vi "T Test (mean).vi"(6 "alternative hypothesis":i32(ring) items=["mean(pop) != mean"=0, "mean(pop) > mean"=1, "mean(pop) < mean"=-1], 9 "significance level":dbl=0.05, 10 "mean":dbl, 11 "sample set":dbl[](array[numeric])) -> (0 "error":i32, 1 "confidence interval":cluster{"low":dbl, "high":dbl}={"low"=0.8260722090132093, "high"=0.8260722090132093} {"high" format="%.6g"; "low" format="%.6g"}, 2 "p value":dbl=0.05 format="%.6g", 3 "reject the null hypothesis":bool, 4 "t test info":T1 {"sample t value" format="%_6g"; "t value" format="%_6g"; "sample se mean" format="%_6g"; "sample std" format="%_6g"; "sample mean" format="%_6g"})   [LabVIEW 2017, in "NI_Gmath.lvlib"]
doc: "See pages 278+ from Applied Statistics and Probability for Engineers (Montgomery) - 3rd Edition."
uses:
  NI_Gmath.lvlib
  st_t_control.ctl
  NI_AALBase.lvlib
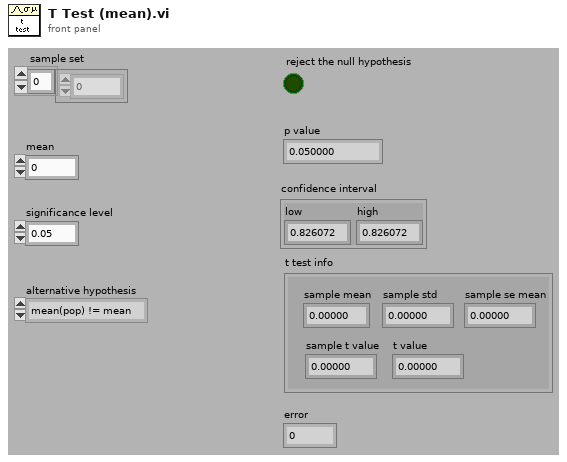
[diagram p1: front panel]
types:
  T1 = typedef "NI_Gmath.lvlib/st_t_control.ctl" = cluster{"sample mean":dbl, "sample std":dbl, "sample se mean":dbl, "sample t value":dbl, "t value":dbl}
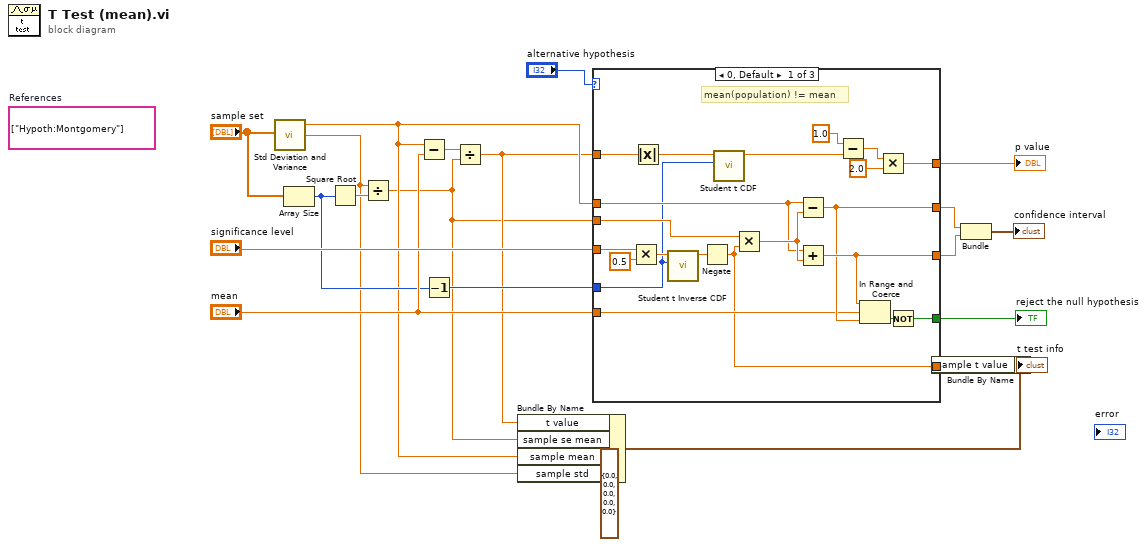
[diagram p0: block diagram]
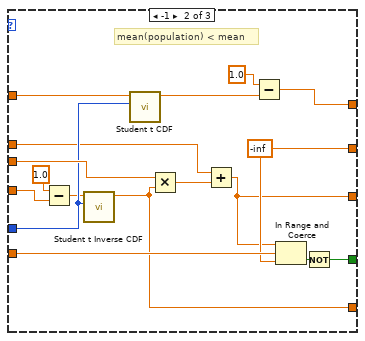
[diagram p2: hidden frame]
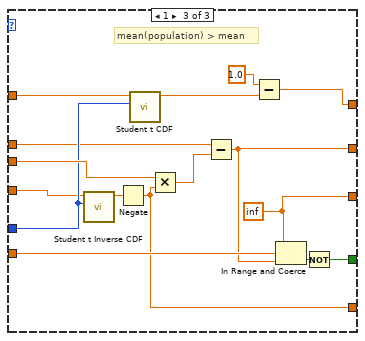
[diagram p3: hidden frame]
diagram:
  (unwired) string[] ["Hypoth:Montgomery"]  # References
  n1 = call "Std Deviation and Variance.vi"("X"="sample set") -> ("mean"=w7:dbl, "standard deviation"=w8:dbl)  [unwired: 1 in, 1 out]
  n2 = Array Size(array="sample set") -> (size(s)=w9:i32)
  n3 = Square Root(x=w9) -> (sqrt(x)=w10:dbl)
  n4 = Divide(x=w8, y=w10) -> (x/y=w5:dbl)
  n5 = Subtract(x=w7, y="mean") -> (x-y=w20:dbl)
  n6 = Decrement(x=w9) -> (x-1=w17:i32)
  n7 = Divide(x=w20, y=w5) -> (x/y=w6:dbl)
  n8 = Bundle By Name(cluster=T1 {"sample mean"=0.0, "sample std"=0.0, "sample se mean"=0.0, "sample t value"=0.0, "t value"=0.0} ("t test info"), "t value"=w6, "sample se mean"=w5, "sample mean"=w7, "sample std"=w8) -> (w4:T1)
  n9 = case shown="0, Default" "alternative hypothesis" {
    tunnel: "significance level" -> [w41 w48 w66]
    tunnel: w17 -> [w30 w55 w70]
    tunnel: w5 -> [w40 w59 w75]
    tunnel: [w36 w43 w63] -> w16
    tunnel: [w35 w44 w64] -> w15
    tunnel: [w33 w56 w72] -> w14
    tunnel: "mean" -> [w32 w51 w71]
    tunnel: w7 -> [w31 w50 w65]
    tunnel: w6 -> [w29 w45 w69]
    tunnel: [w24 w52 w62] -> w11
    tunnel: [w23 w46 w60] -> w2
    frame 0, Default {
      # "mean(population) != mean"
      n10 = Multiply(x=w41, y=0.5) -> (x*y=w37:dbl)
      n11 = Absolute Value(x=w29) -> (abs(x)=w22:dbl)
      n12 = call "Student t Inverse CDF.vi"("k degrees of freedom"=w30, "cdf(x)"=w37) -> ("x"=w38:dbl)  [unwired: 8 in, 1 out]
      n13 = Negate(x=w38) -> (-x=w23:dbl)
      n14 = call "Student t CDF.vi"("k degrees of freedom"=w30, "x"=w22) -> ("cdf(x)"=w27:dbl)  [unwired: 7 in, 2 out]
      n15 = Multiply(x=w40, y=w23) -> (x*y=w39:dbl)
      n16 = Subtract(x=w31, y=w39) -> (x-y=w35:dbl)
      n17 = Add(x=w31, y=w39) -> (x+y=w36:dbl)
      n18 = Subtract(x=1.0, y=w27) -> (x-y=w25:dbl)
      n19 = In Range and Coerce(upper limit=w36, x=w32, lower limit=w35) -> (In Range?=w34:bool)  [unwired: 1 out]
      n20 = Multiply(x=w25, y=2.0) -> (x*y=w24:dbl)
      n21 = Not(x=w34) -> (.not. x?=w33:bool)
    }
    frame -1 {
      w44 = -inf ("lower limit")
      # "mean(population) < mean"
      n22 = Subtract(x=1.0, y=w48) -> (x-y=w47:dbl)
      n23 = call "Student t Inverse CDF.vi"("k degrees of freedom"=w55, "cdf(x)"=w47) -> ("x"=w46:dbl)  [unwired: 8 in, 1 out]
      n24 = call "Student t CDF.vi"("k degrees of freedom"=w55, "x"=w45) -> ("cdf(x)"=w53:dbl)  [unwired: 7 in, 2 out]
      n25 = Multiply(x=w59, y=w46) -> (x*y=w58:dbl)
      n26 = Add(x=w50, y=w58) -> (x+y=w43:dbl)
      n27 = Subtract(x=1.0, y=w53) -> (x-y=w52:dbl)
      n28 = In Range and Coerce(upper limit=w43, x=w51, lower limit=w44) -> (In Range?=w57:bool)  [unwired: 1 out]
      n29 = Not(x=w57) -> (.not. x?=w56:bool)
    }
    frame 1 {
      w63 = inf
      # "mean(population) > mean"
      n30 = call "Student t Inverse CDF.vi"("k degrees of freedom"=w70, "cdf(x)"=w66) -> ("x"=w61:dbl)  [unwired: 8 in, 1 out]
      n31 = Negate(x=w61) -> (-x=w60:dbl)
      n32 = call "Student t CDF.vi"("k degrees of freedom"=w70, "x"=w69) -> ("cdf(x)"=w67:dbl)  [unwired: 7 in, 2 out]
      n33 = Multiply(x=w75, y=w60) -> (x*y=w74:dbl)
      n34 = Subtract(x=w65, y=w74) -> (x-y=w64:dbl)
      n35 = Subtract(x=1.0, y=w67) -> (x-y=w62:dbl)
      n36 = In Range and Coerce(upper limit=w63, x=w71, lower limit=w64) -> (In Range?=w73:bool)  [unwired: 1 out]
      n37 = Not(x=w73) -> (.not. x?=w72:bool)
    }
  }
  "reject the null hypothesis" <- w14
  "p value" <- w11
  n38 = Bundle By Name(cluster=w4, "sample t value"=w2) -> (→"t test info":T1)
  n39 = Bundle("lower limit"=w15, w16) -> (→"confidence interval":cluster{"lower limit":dbl, dbl})  [unwired: 1 in]
